vi "get Origin.vi"(11 "Camera in":refnum<class "Camera.lvclass">) -> (3 "Origin":refnum<class "Vector 2D.lvclass">)   [LabVIEW 2021, in "Camera.lvclass"]
uses:
  Camera.lvclass
  Re-use Libraries/Vector 2D/Vector 2D.lvclass
  Camera.lvclass/Camera.ctl
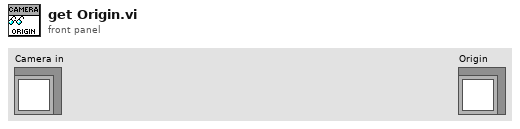
[diagram p1: front panel]
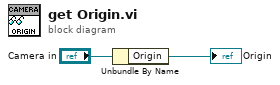
[diagram p0: block diagram]
diagram:
  n1 = Unbundle By Name("Camera in") -> ("Origin"=→"Origin":refnum<class "Vector 2D.lvclass">)
